vi "Find Child Attributes.vi"(7 "Actor in":refnum<class "Actor.lvclass">, 10 "Alias":string) -> (0 "Error out":errorcluster, 2 "Child Attributes":refnum<class "Attributes.lvclass">)   [LabVIEW 2020, in "jettl.lvlib"]
uses:
  jettl.lvlib
  Attributes/Attributes.lvclass
  Actor/Actor.lvclass
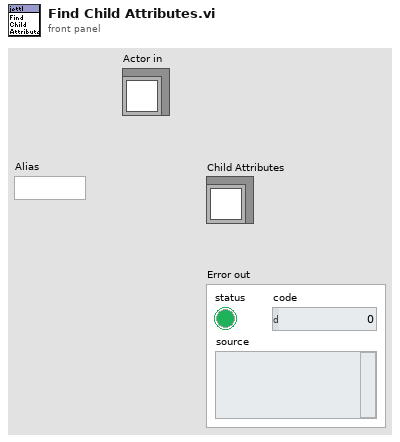
[diagram p1: front panel]
types:
  T1 = typedef "jettl.lvlib/All Child Attributes.ctl" = map{string, refnum<class "Attributes.lvclass">}
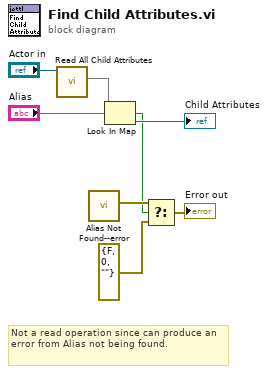
[diagram p0: block diagram]
diagram:
  # "Not a read operation since can produce an error from Alias not being found."
  n1 = call-dynamic "Read All Child Attributes.vi"("Actor in"="Actor in") -> ("All Child Attributes"=w3:T1)  [unwired: 10 in]
  n2 = call "Alias Not Found--error.vi"() -> ("Error"=w7:errorcluster)  [unwired: 11 in]
  n3 = Look In Map(map=w3, key="Alias") -> (key not found?=w1:bool, value=→"Child Attributes":refnum<class "Attributes.lvclass">)  [unwired: 1 in]
  n4 = Select(t=w7, s=w1, f=errorcluster {"status"=FALSE, "code"=0, "source"=""}) -> (s? t:f=→"Error out":errorcluster)
